vi "Initialize.vi"(0 "Yokogawa WT500 in":refnum<class "Yokogawa WT500.lvclass">, 7 "Reset (T: Reset)":bool=TRUE, 9 "ID Query (T: Check)":bool=TRUE, 11 "error in (no error)":errorcluster) -> (4 "Yokogawa WT500 out":refnum<class "Yokogawa WT500.lvclass">, 6 "VISA resource name":refnum<visa-resource-name>, 15 "error out":errorcluster)   [LabVIEW 2013, in "Universal Power Meter.lvlib" / "Yokogawa WT500.lvlib" / "Yokogawa WT500.lvclass"]
uses:
  Yokogawa WT500.lvclass
  Universal Power Meter class/Universal Power Meter.lvclass
  <instrlib>/ykwt500/ykwt500.llb/YKWT500 Read Numeric (Normal).vi
panel:
  out "Array":i32[](array[numeric])
  out "Actual output":u16[][][](array[numeric])
  out "Element (0: All)":u16
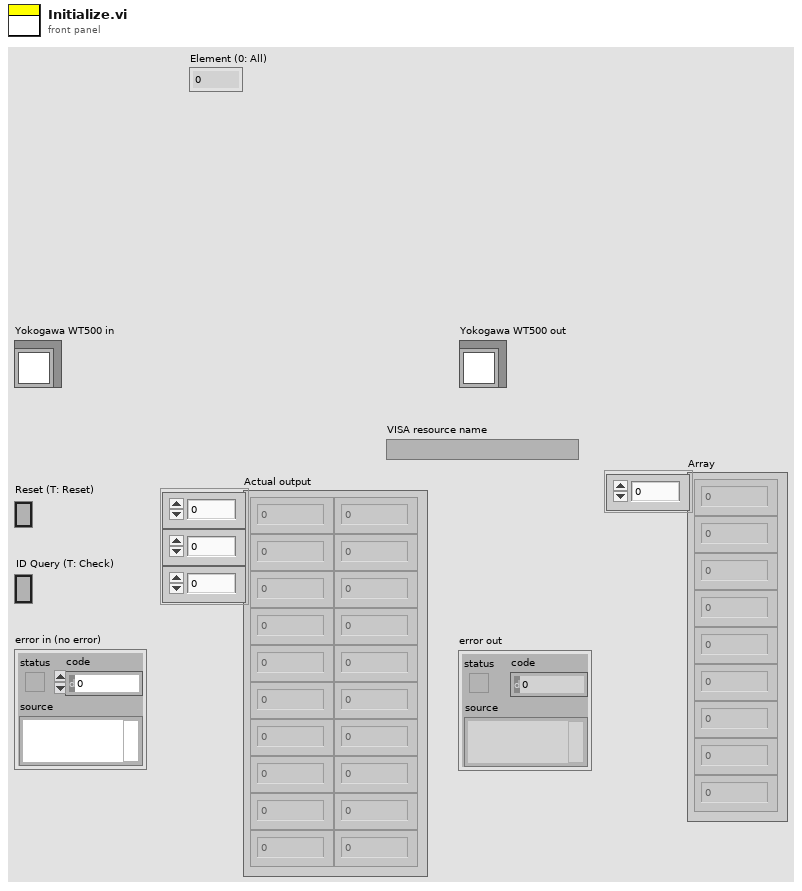
[diagram p1: front panel]
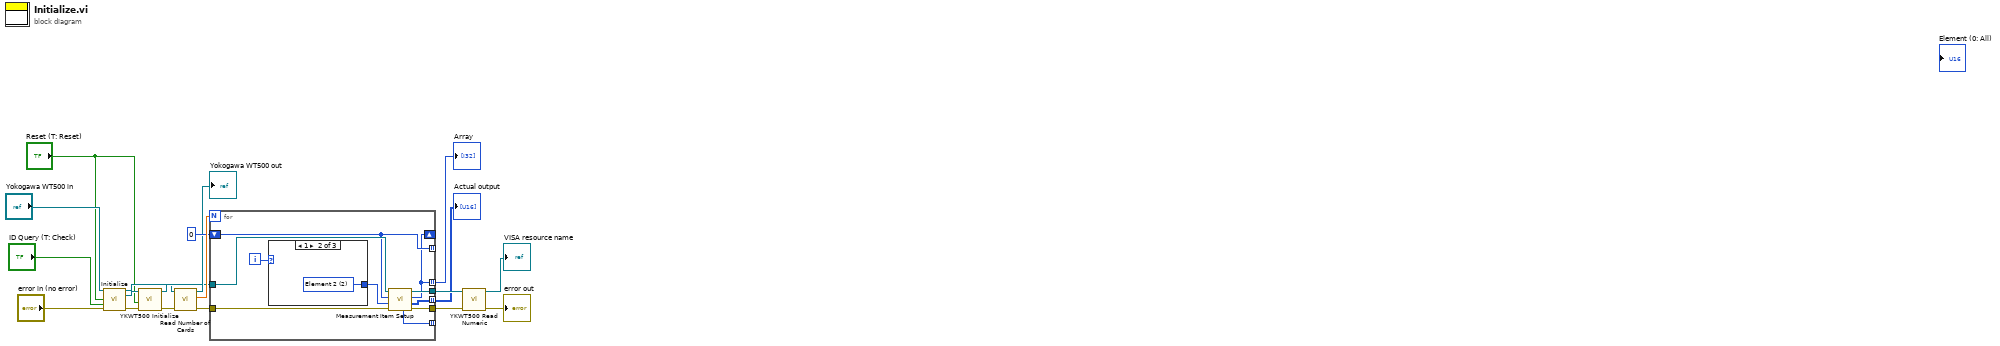
[diagram p0: block diagram]
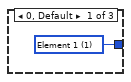
[diagram p2: hidden frame]
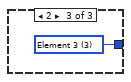
[diagram p3: hidden frame]
diagram:
  n1 = call-parent "Initialize.vi"("Universal Power Meter in"="Yokogawa WT500 in", "Reset (T: Reset)"="Reset (T: Reset)", "ID Query (T: Check)"="ID Query (T: Check)", "error in (no error)"="error in (no error)") -> ("Universal Power Meter out"=w2:refnum<class "Yokogawa WT500.lvclass">, "VISA resource name"=w6:refnum<visa-resource-name>, "error out"=w5:errorcluster)  [unwired: 9 in]
  n2 = call <instrlib>:"YKWT500 Initialize.vi"("error in (no error)"=w5, "Reset (True)"="Reset (T: Reset)", "VISA resource name"=w6) -> ("error out"=w4:errorcluster, "VISA resource name out"=w3:refnum<visa-resource-name>)  [unwired: 7 in]
  n3 = call-dynamic "Read Number of Cards.vi"("error in (no error)"=w4, "Generic Instrument in"=w2) -> ("error out"=w18:errorcluster, "Number of Cards"=w14:dbl, "Generic Instrument out"=→"Yokogawa WT500 out":refnum<class "Yokogawa WT500.lvclass">)  [unwired: 7 in]
  n4 = for {
    N: w14 -> [_]
    tunnel: w3 -> [w29]
    tunnel: w18 -> [w28]
    tunnel: [w27] -> w17
    tunnel: [w26] -> w15
    tunnel: [w25] -> w8 mode=indexing
    shift-right: [w20] -> _
    shift-left: 0 ("i-j") -> [w21]
    tunnel: [w22] -> _ mode=indexing
    tunnel: [w21] -> _ mode=indexing
    tunnel: [w20] -> w7 mode=indexing
    i -> [w23]
    n5 = case shown="1" w23 {
      tunnel: [w30 w31 w32] -> w24
      frame 0, Default {
        w30 = u16 1 items=["All", "Element 1", "Element 2", "Element 3", "Sigma"] ("Element (0: All)")
      }
      frame 1 {
        w31 = u16 2 items=["All", "Element 1", "Element 2", "Element 3", "Sigma"] ("Element (0: All)")
      }
      frame 2 {
        w32 = u16 3 items=["All", "Element 1", "Element 2", "Element 3", "Sigma"] ("Element (0: All)")
      }
    }
    n6 = call "Measurement Item Setup.vi"("error in (no error)"=w28, "Element (0: All)"=w24, "i-j"=w21, "VISA Refnum in"=w29) -> ("error out"=w26:errorcluster, "Actual output"=w25:u16[][], "i-j 2"=w20:i32, "VISA Refnum out"=w27:refnum<visa-resource-name>, "position"=w22:i32[])  [unwired: 3 in]
  }
  "Actual output" <- w8
  "Array" <- w7
  n7 = call-poly <instrlib>:"YKWT500 Read Numeric.vi"("error in (no error)"=w15, "VISA resource name"=w17) -> ("error out"=→"error out":errorcluster, "VISA resource name out"=→"VISA resource name":refnum<visa-resource-name>)  [unwired: 7 in, 1 out]
